vi "TempConfigurationSubVIold.vi"(8 "error in":errorcluster, 10 "Sim?":bool, 11 "physical channels":tag) -> (0 "error out":errorcluster, 3 "temperature task out":refnum<k21> caption="task out")   [LabVIEW 2015]
uses:
  <vilib>/DAQmx/configure/timing.llb/DAQmx Timing (Sample Clock).vi
  <vilib>/DAQmx/create/channels.llb/DAQmx Create Channel (AI-Voltage-Basic).vi
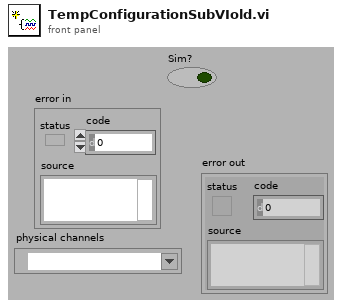
[diagram p1: front panel]
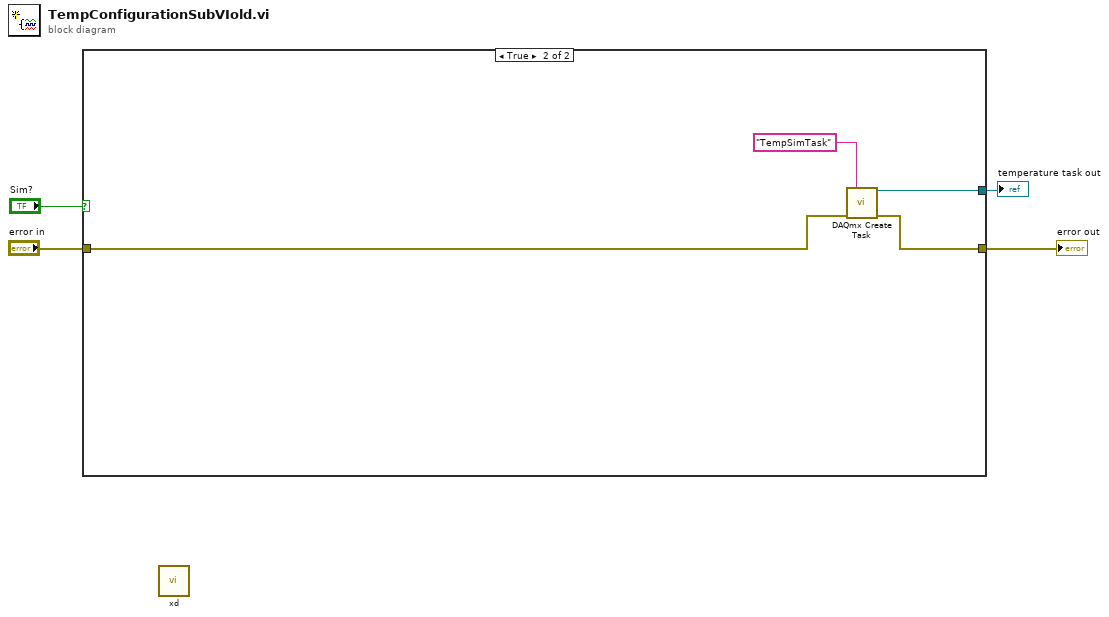
[diagram p0: block diagram]
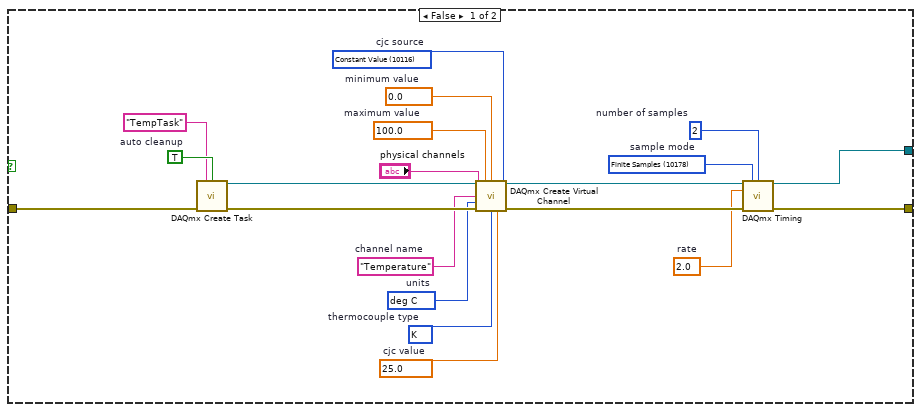
[diagram p2: hidden frame]
diagram:
  n1 = case shown="True" "Sim?" {
    tunnel: "error in" -> [w24 w25]
    tunnel: [w12 w27] -> w3
    tunnel: [w5 w26] -> w1
    frame False {
      w8 = 10178 items=["Finite Samples"=10178, "Continuous Samples"=10123, "Hardware Timed Single Point"=12522]  # sample mode
      w9 = 2  # number of samples
      w10 = 2.0  # rate
      w13 = 10116 items=["Built-In"=10200, "Constant Value"=10116, "Channel"=10113]  # cjc source
      w15 = 25.0  # cjc value
      w16 = 10073 items=["J"=10072, "K"=10073, "N"=10077, "R"=10082, "S"=10085, "T"=10086, "B"=10047, "E"=10055]  # thermocouple type
      w17 = 10143 items=["deg C"=10143, "deg F"=10144, "Kelvins"=10325, "deg R"=10145, "From Custom Scale"=10065]  # units
      w14 = "Temperature"  # channel name
      w19 = 0.0  # minimum value
      w20 = 100.0  # maximum value
      w22 = TRUE  # auto cleanup
      n2 = call <vilib>:"DAQmx Create Task.vi"("new task name"="TempTask", "auto cleanup"=w22, "error in"=w24) -> ("task out"=w21:refnum<k21>, "error out"=w23:errorcluster)  [unwired: 11 in]
      n3 = call-poly <vilib>:"DAQmx Create Virtual Channel.vi"("task in"=w21, "maximum value"=w20, "minimum value"=w19, "physical channels"="physical channels", 6:w13, "name to assign"=w14, "units"=w17, "error in"=w23, 13:w16, 14:w15) -> ("task out"=w11:refnum<k21>, "error out"=w18:errorcluster)  [unwired: 4 in]
      n4 = call-poly <vilib>:"DAQmx Timing.vi"("task/channels in"=w11, "sample mode"=w8, "samples per channel"=w9, "rate"=w10, "error in"=w18) -> ("task out"=w12:refnum<k21>, "error out"=w5:errorcluster)  [unwired: 9 in]
    }
    frame True {
      n5 = call <vilib>:"DAQmx Create Task.vi"("new task name"="TempSimTask", "error in"=w25) -> ("task out"=w27:refnum<k21>, "error out"=w26:errorcluster)  [unwired: 12 in]
    }
  }
  "temperature task out" <- w3
  "error out" <- w1
  n6 = call "xd.vi"() -> ()  [unwired: 10 in, 2 out]
